vi "Turn On.vi"(8 "error in (no error)":errorcluster, 11 "Switchable Device in":refnum<class "Switchable Device.lvclass">) -> (0 "error out":errorcluster, 3 "Switchable Device out":refnum<class "Switchable Device.lvclass">)   [LabVIEW 2018, in "Switchable Device.lvclass"]
uses:
  Switchable Device.lvclass
  Switchable Device.lvclass/Switchable Device.ctl
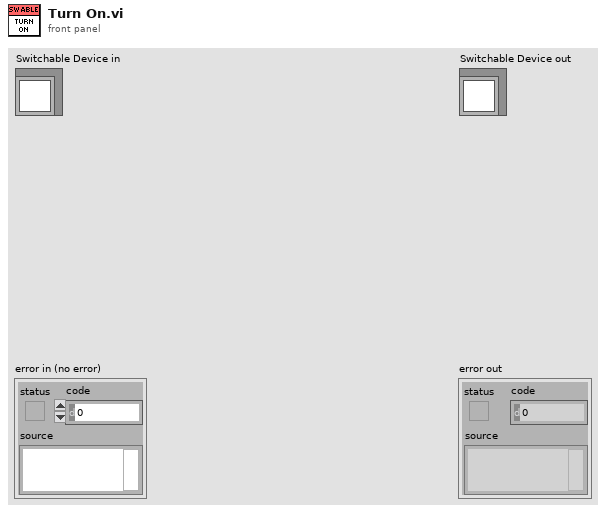
[diagram p1: front panel]
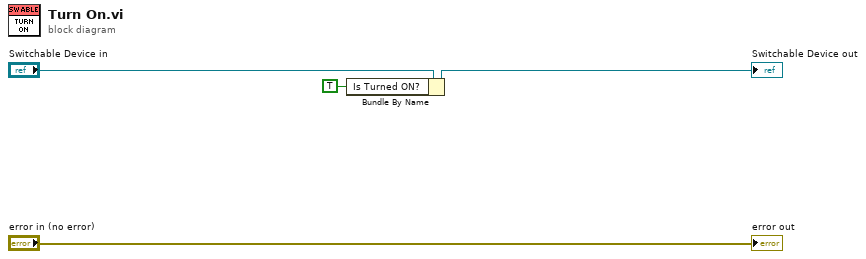
[diagram p0: block diagram]
diagram:
  n1 = Bundle By Name(cluster="Switchable Device in", "Is Turned ON?"=TRUE) -> (→"Switchable Device out":refnum<class "Switchable Device.lvclass">)
  "error out" <- "error in (no error)"
